vi "Patch data export-Initialise montage gen.vi"(0 "ExperimentPath":path, 1 "First init.":bool, 2 "Output file path":path=path "C:/Users/Teo/Desktop/UCL Datasets/160915_13_48_57 FunctAcq-6 patches", 5 "Frames Per Second":u32=30, 7 "Channel":i32, 9 "Number of rows to generate":i32=6, 11 "error in (no error)":errorcluster) -> (3 "Experiment Parameters":T4, 4 "Image ref (Montage)":T3, 6 "Coordinates of montage positions":cluster{"X\n\nY":i32[]}[](array[cluster]), 8 "TDMS references(All Trials)":refnum<k34>[](array[refnum]), 10 "Frames info":T2, 13 "Cancel":bool, 14 "AVI Refnum":T1, 15 "error out":errorcluster)   [LabVIEW 2017]
uses:
  User Interface/Visualisation/Patch-Vol video generator/Typedefs/Experiment Parameters.ctl
  <vilib>/vision/Image Controls.llb/IMAQ Image.ctl
  <vilib>/vision/Avi.llb/IMAQ AVI2 Refnum.ctl
  User Interface/Visualisation/Patch-Vol video generator/Globals/gl_8-bit montage window ctrl refs.vi
panel:
  in  "Peak value in dataset (I16)":dbl=17960.0 format="%#_13g"
  out "max value":dbl
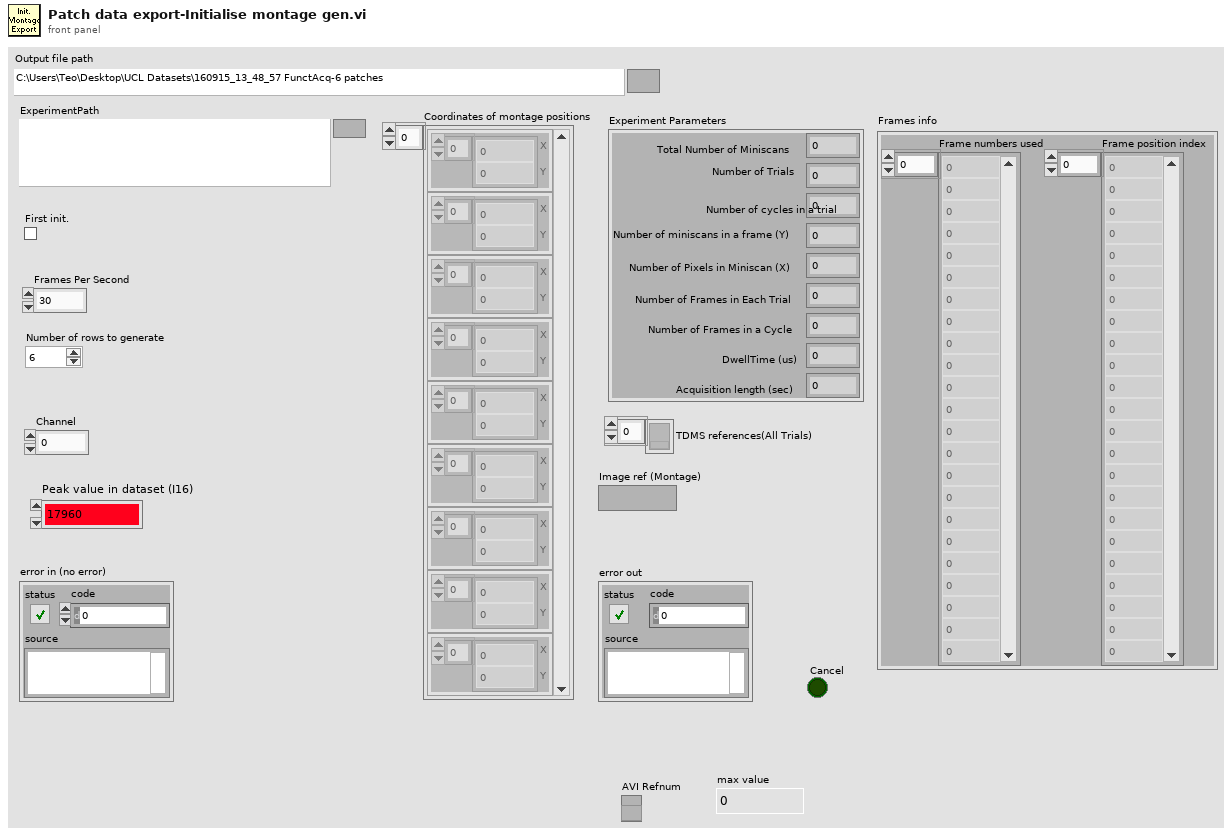
[diagram p1: front panel]
types:
  T1 = typedef "IMAQ AVI2 Refnum.ctl" = refnum<k20>
  T2 = cluster{"Frame numbers used":i32[], "Frame position index":i32[]}
  T3 = typedef "IMAQ Image.ctl" = refnum<image>
  T4 = typedef "Experiment Parameters.ctl" = cluster{"Total Number of Miniscans":i32, "Number of Trials":i32, "Number of cycles in a trial":i32, "Number of miniscans in a frame (Y)":i32, "Number of Pixels in Miniscan (X)":i32, "Number of Frames in Each Trial":i32, "Number of Frames in a Cycle":i32, "DwellTime (us)":dbl, "Acquisition length (sec)":dbl}
  T5 = cluster{"Number of rows to generate":i32, "Number of columns to generate":i32}
  T6 = typedef "8-bit video export window ctrl refs.ctl" = cluster{"This VI":refnum<vi>, "Add speed data":refnum<vi>, "Add camera videos":refnum<vi>, "Stop button":refnum<vi>, "Camera Video Adjustments":refnum<vi>, "Microscope Image Adjustments":refnum<vi>, "Execute":refnum<vi>, "Codec":refnum<vi>, "Channel to load":refnum<vi>, "Speed graph behaviour":refnum<vi>, "Include speed graph":refnum<vi>, "Number of rows to generate":refnum<vi>, "Path":refnum<vi>}
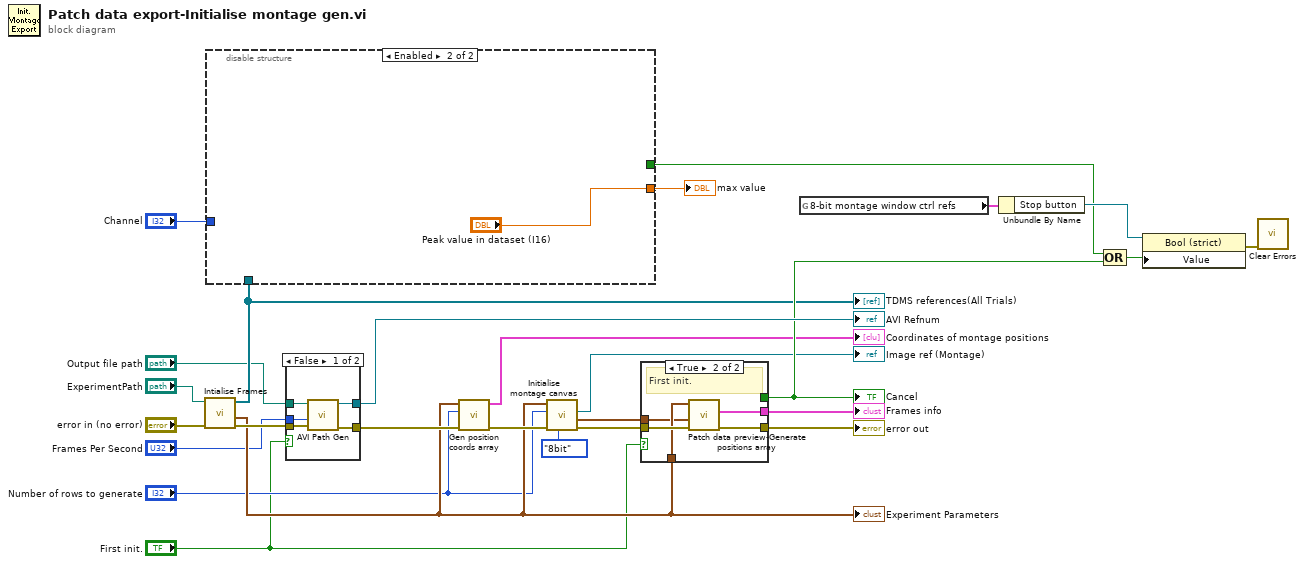
[diagram p0: block diagram]
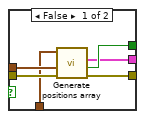
[diagram p3: hidden frame]
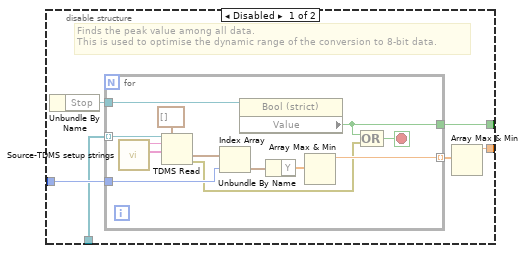
[diagram p4: hidden frame]
diagram:
  n1 = call "Intialise Frames.vi"("error in (no error)"="error in (no error)", "ExperimentPath"="ExperimentPath") -> ("error out"=w27:errorcluster, "Experiment Parameters"=w8:T4, "TDMS references(All Trials)"=w7:refnum<k34>[])  [unwired: 6 in, 1 out]
  "Experiment Parameters" <- w8
  "TDMS references(All Trials)" <- w7
  n2 = disable-structure shown="Enabled" {
    disable-tunnel: "Channel" -> [w33 _]
    disable-tunnel: w7 -> [w32 _]
    disable-tunnel: [w31 "Peak value in dataset (I16)"] -> w20
    disable-tunnel: [w28 _] -> w16
    frame Disabled {
      # "Finds the peak value among all data.\nThis is used to optimise the dynamic range of the conversion to 8-bit data."
      n3 = Unbundle By Name() -> ("Stop"=w29:refnum<vi>)  [unwired: 1 in]
      n4 = for {
        tunnel: [w40] -> w30 mode=indexing
        tunnel: w32 -> [w39] mode=indexing
        tunnel: w33 -> [w38]
        tunnel: w29 -> [w37]
        tunnel: [w34] -> w28
        stop <- w35 stop-if-true
        n5 = call "Source-TDMS setup strings.vi"() -> ("Functional imaging TDMS channel names array"=w43:string[], "TDMS group name"=w44:string)  [unwired: 10 in]
        n6 = TDMS Read(0:w39, 5:w44, 7:w43, 12:waveform(dbl)[] [] ("data type")) -> (10:w45:waveform(dbl)[], 15:w36:errorcluster)  [unwired: 4 in, 4 out]
        n7 = Index Array(array=w45, index=w38) -> (element=w46:waveform(dbl))
        n8 = property class="Bool (strict)"(reference=w37) -> ("Value"=w34:bool)  [unwired: 1 in, 2 out]
        n9 = Unbundle By Name(w46) -> ("Y"=w41:dbl[])
        n10 = Array Max & Min(array=w41) -> (max value=w40:dbl)  [unwired: 3 out]
        n11 = Compound Arithmetic op=OR(w34, w36) -> (w35:bool)
      }
      n12 = Array Max & Min(array=w30) -> (max value=w31:dbl)  [unwired: 3 out]
    }
    frame Enabled {
    }
  }
  "max value" <- w20
  n13 = case shown="False" "First init." {
    tunnel: w27 -> [w52 w53]
    tunnel: [w51 _] -> w26
    tunnel: [w50 w53] -> w25
    tunnel: "Frames Per Second" -> [w49 _]
    tunnel: "Output file path" -> [w48 _]
    frame False {
      n14 = call "AVI Path Gen.vi"("error in (no error)"=w52, "Frames Per Second"=w49, "Output file path"=w48) -> ("error out"=w50:errorcluster, "AVI Refnum"=w51:T1)  [unwired: 6 in, 1 out]
    }
    frame True {
      # "First init."
    }
  }
  "AVI Refnum" <- w26
  n15 = call "Gen position coords array.vi"("Error in"=w25, "Number of rows to generate"="Number of rows to generate", "Experiment Parameters"=w8) -> ("error out"=w24:errorcluster, "Coordinates of montage positions"=→"Coordinates of montage positions":cluster{"X\n\nY":i32[]}[])  [unwired: 7 in]
  n16 = call "Initialise montage canvas.vi"("Image bitness"=enum16{"8bit", "16bit"}."8bit", "Error in"=w24, "Number of rows to generate"="Number of rows to generate", "Experiment Parameters"=w8) -> ("error out"=w23:errorcluster, "Rows/Columns"=w22:T5, "U8 Image ref (Montage)"=→"Image ref (Montage)":T3)  [unwired: 4 in, 1 out]
  n17 = case shown="True" "First init." {
    tunnel: w23 -> [w59 w64]
    tunnel: w22 -> [w58 w60]
    tunnel: [w57 _] -> w18
    tunnel: [w56 w62] -> w10
    tunnel: [w55 w63] -> w9
    tunnel: w8 -> [w54 w61]
    frame False {
      n18 = call "Generate positions array.vi"("Error in"=w59, "Rows/Columns"=w58, "Experiment Parameters"=w54) -> ("error out"=w55:errorcluster, "Cancel"=w57:bool, "Frames info"=w56:T2)  [unwired: 6 in]
    }
    frame True {
      # "First init."
      n19 = call "Patch data preview-Generate positions array.vi"("Error in"=w64, "Rows/Columns"=w60, "Experiment Parameters"=w61) -> ("error out"=w63:errorcluster, "Frames info"=w62:T2)  [unwired: 7 in]
    }
  }
  "error out" <- w9
  "Frames info" <- w10
  "Cancel" <- w18
  n20 = global read "gl_8-bit montage window ctrl refs.vi" "8-bit montage window ctrl refs"() -> (w15:T6)
  n21 = Unbundle By Name(w15) -> ("Stop button"=w19:refnum<vi>)
  n22 = Compound Arithmetic op=OR(w16, w18) -> (w17:bool)
  n23 = property class="Bool (strict)"(reference=w19, "Value"=w17) -> (error out=w14:errorcluster)  [unwired: 1 in, 1 out]
  n24 = call <vilib>:"Clear Errors.vi"("error in (no error)"=w14) -> ()  [unwired: 5 in, 2 out]
